vi "Write Lockin Digitizer Configuration.vi"(8 "error in (no error)":errorcluster, 10 "Configuration":T1={"Post-trigger delay"=0.01, "Post-trigger duration"=0.1, "Rate"=1000000.0, "Ranges"=[10.0], "Re-name channels"=[], "Active channels"="0:1", "External clock"=FALSE, "Frequencies"=[], "Time \nconstants"=[], "Output \namplitudes"=[], "Lock-in #"=[]} {"Output \namplitudes" format="%#_6pV"; "Time \nconstants" format="%#_6ps"; "Frequencies" format="%#_6pHz"; "Rate" format="%#_8pHz"; "Post-trigger duration" format="%#_6ps"; "Post-trigger delay" format="%#_6ps"; "Ranges" format="%#_6pV"}, 11 "Lockin Digitizer in":refnum<class "Lockin Digitizer.lvclass">) -> (0 "error out":errorcluster, 3 "Lockin Digitizer out":refnum<class "Lockin Digitizer.lvclass">)   [LabVIEW 2021, in "Lockin Digitizer.lvclass"]
uses:
  Lockin Digitizer.lvclass
  Lockin Digitizer.lvclass/Lockin Digitizer.ctl
  NHMFL_Core/Libraries/Instruments/Lockin Digitizer Driver/Lockin Digitizer Configuration.ctl
panel:
  # "Digitizer config"
  # "Lock-in config"
  # "#0\n\n#1"
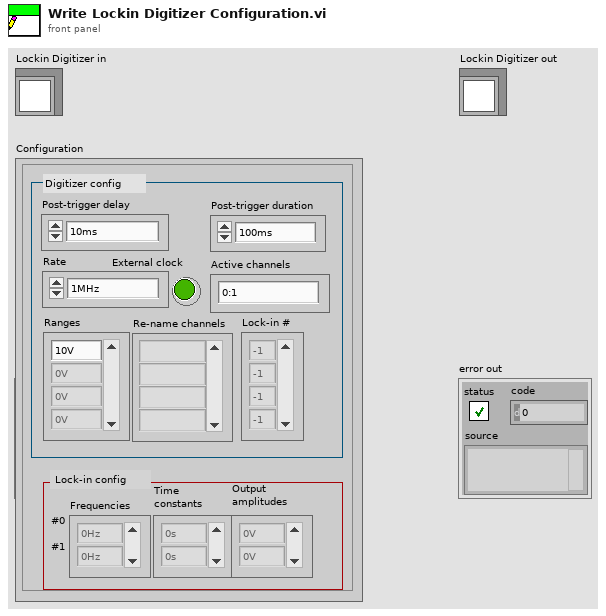
[diagram p1: front panel]
types:
  T1 = typedef "Lockin Digitizer Configuration.ctl" = cluster{"Post-trigger delay":dbl, "Post-trigger duration":dbl, "Rate":dbl, "Ranges":dbl[], "Re-name channels":string[], "Active channels":string, "External clock":bool, "Frequencies":dbl[], "Time \nconstants":dbl[], "Output \namplitudes":dbl[], "Lock-in #":i32[]}
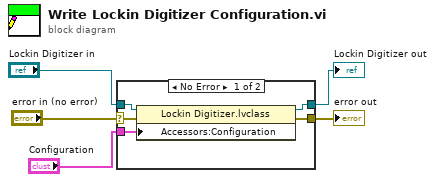
[diagram p0: block diagram]
diagram:
  n1 = case shown="No Error" "error in (no error)" {
    selector: "error in (no error)" -> [w8 w11]
    tunnel: [w7 w11] -> w4
    tunnel: [w6 w12] -> w2
    tunnel: "Lockin Digitizer in" -> [w10 w12]
    tunnel: "Configuration" -> [w9 _]
    frame No Error {
      n2 = property class="Lockin Digitizer.lvclass"(reference=w10, error in=w8, "Accessors:Configuration"=w9) -> (reference out=w6:refnum<class "Lockin Digitizer.lvclass">, error out=w7:errorcluster)
    }
    frame Error {
    }
  }
  "error out" <- w4
  "Lockin Digitizer out" <- w2
